vi "PrefDialog.vi"(8 "error in (no error)":errorcluster, 11 "MyPluginsBase in":refnum<class "ChromaPowerSupply.lvclass">) -> (0 "error out":errorcluster, 1 "Save As":bool, 2 "Changed":bool, 3 "MyPluginsBase out":refnum<class "ChromaPowerSupply.lvclass">)   [LabVIEW 2018, in "AcPwrPlugins.lvlib" / "ChromaPowerSupply.lvclass"]
doc: "This VI displays the prior instruments properties and allows a user to change the instrument properties and save these new set properties to the same location on disk or in a new location with a new name called \"Type\"."
uses:
  ChromaPowerSupply.lvclass
  C:/Program Files (x86)/National Instruments/LabVIEW 2018/user.lib/NIST/BaseClasses/BasePlugin_class/BasePlugin.lvclass
  C:/Users/Public/Projects/ICDAS/NistPluggableModules/AcPwr/AcPwrPlugins/AcPwrBaseClass/AcPwrBase.lvclass
  TypeDefs/Measurements.ctl
  AcPwrBaseClass/TypeDefs/BaseMeasurements.ctl
  ChromaAcLoad/TypeDefs/MeasurementType.ctl
  TypeDefs/Device(s)Settings.ctl
  <userlib>/NIST/BaseClasses/BasePlugin_class/BasePlugin.lvclass/BasePlugin.ctl
  AcPwrBaseClass/AcPwrBase.lvclass/AcPwrBase.ctl
  <userlib>/NIST/BaseClasses/BasePlugin_class/Accessors/Read PluginIniFilePath.vi
  AcPwrBaseClass/Accessors/Read BaseConfig.vi
  AcPwrBaseClass/Accessors/Read BaseMeasurements.vi
  <userlib>/NIST/BaseClasses/BasePlugin_class/Accessors/Write PluginIniFilePath.vi
  <vilib>/Utility/config.llb/NI_LVConfig.lvlib
  AcPwrBaseClass/AcPwrBase.lvclass
  ChromaAcLoad/ChromaAcLoad.lvclass
panel:
  in  "btnSaveAs":bool
  in  "btnSave":bool
  in  "Measurement RefreshTime (ms)":u32
  in  "Device(s)Settings":T1
  in  "BaseMeasurements":T2 {"NHRGridSim Phase" items=["All", "A Phase", "B Phase", "C Phase"]; "NHRDC Measurement Type" items=["Voltage"=1, "Positive Peak Voltage"=2, "Positive Peak Voltage Last Fetch"=4, "Negative Peak Voltage"=8, "Negative Peak Voltage Last Fetch"=16, "Current"=32, "Positive Peak Current"=64, "Positive Peak Current Last Fetch"=128, "Negative Peak Current"=256, "Negative Peak Current Last Fetch"=512, "Power"=1024, "Positive Peak Power"=2048, "Positive Peak Power Last Fetch"=4096, "Negative Peak Power"=8192, "Negative Peak Power Last Fetch"=16384, "Timestamp"=32768, "Charge Time"=65536, "Discharge Time"=131072, "Amp Hour"=262144, "Amp Hour Time"=524288, "Amp Hour Charge"=1048576, "Amp Hour Discharge"=2097152, "Kilo Watt Hour"=4194304, "Kilo Watt Hour Time"=8388608, "Kilo Watt Hour Charge"=16777216, "Kilo Watt Hour Discharge"=33554432, "UUT Temperature"=67108864]; "NHRDC Fetch Method" items=["Aperture", "Immediate"]}
  in  "Measurements":T4
  in  "btnCancel":bool
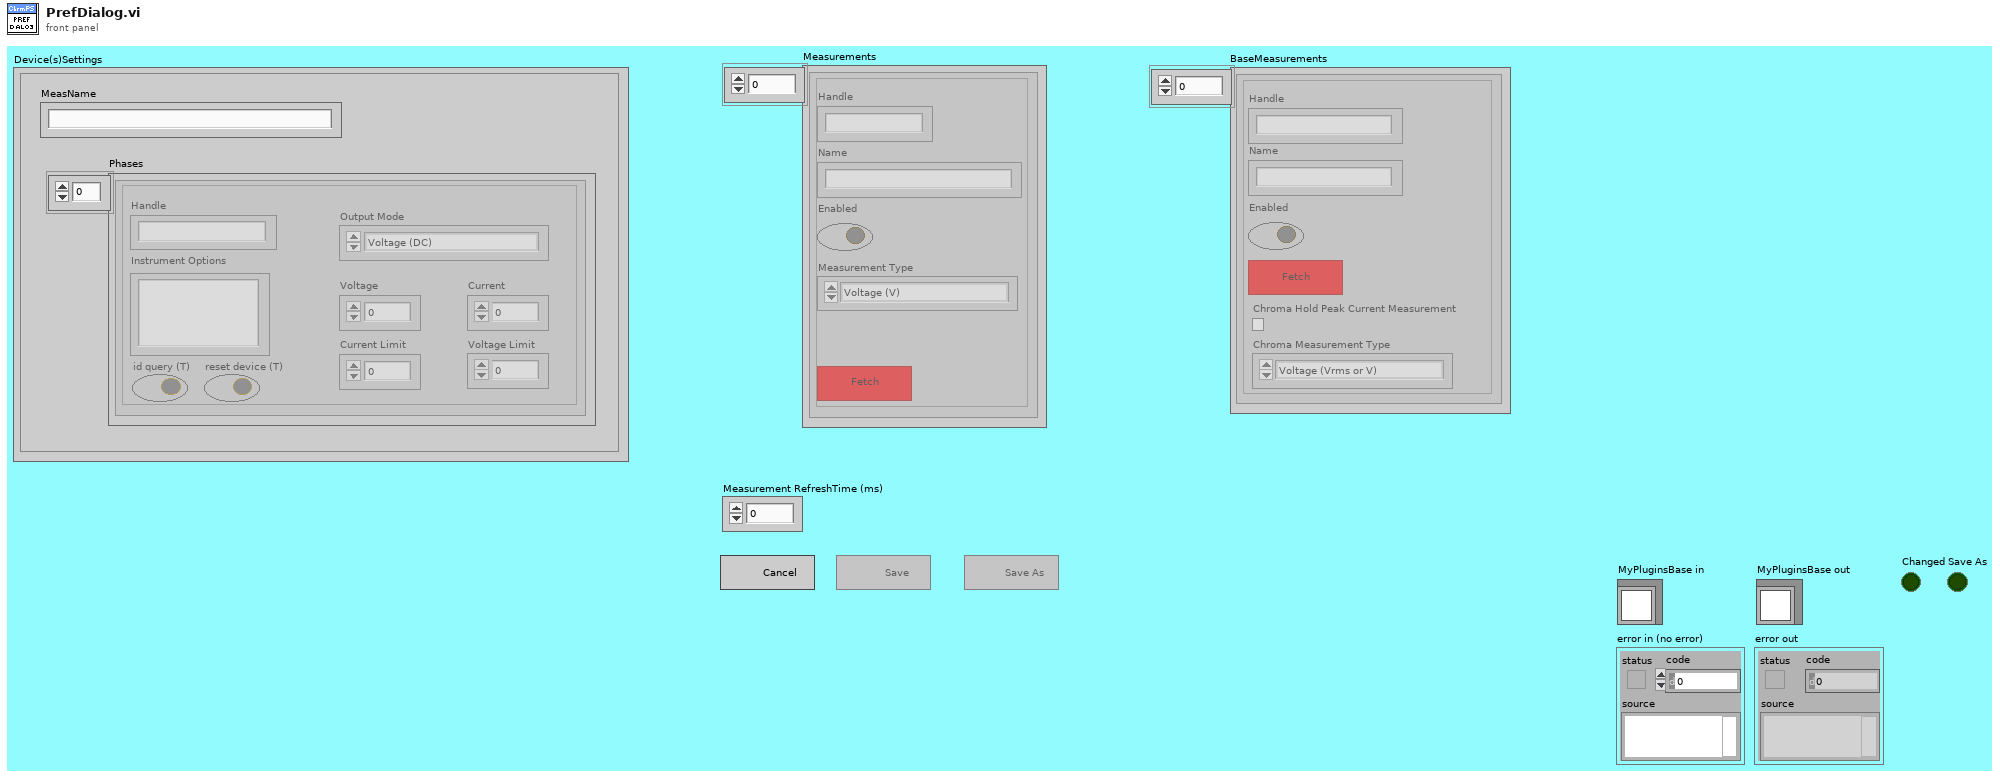
[diagram p1: front panel]
types:
  T1 = typedef "AcPwrPlugins.lvlib/ChromaPowerSupply.lvclass/Device(s)Settings.ctl" = cluster{"Phases":cluster{"Handle":string, "Instrument Options":string, "id query (T)":bool, "reset device (T)":bool, "Timing":cluster{"TimingOn":enum16{""}, "Hours":u32, "Minutes":u32, "Seconds":dbl, "CutoffVoltage":dbl}, "Connected":bool, "Output Mode":enum16{"Voltage (DC)", "Current (DC)"}, "Voltage":dbl, "Current":dbl, "Voltage Limit":dbl, "Current Limit":dbl}[], "MeasName":string}
  T2 = typedef "AcPwrPlugins.lvlib/AcPwrBase.lvclass/BaseMeasurements.ctl" = cluster{"Handle":string, "Name":string, "Enabled":bool, "Measurement Value":dbl, "btnMeasFetch":bool, "Chroma Hold Peak Current Measurement":bool, "Chroma Measurement Type":T3, "Chroma Protection Status String":string, "NHRDC Fetch Method":i32, "NHRDC Fetch Time (s)":sgl, "NHRDC Measurement Type":i32, "NHRGridSim Measurement Type ":enum16{"Average Current", "Max Current", "Min Current", "Average Voltage", "Max Voltage", "Min Voltage", "Average True Power", "Max True Power", "Min True Power", "Average Apparent Power", "Max Apparent Power", "Min Apparent Power", "Power Factor", "Crest Factor"}, "NHRGridSim Phase ":i32, "PPS Measurement Type ":enum16{"Voltage RMS L-N", "Voltage RMS L-L", "Frequency", "Current RMS", "Current Peak", "Crest Factor", "Power Factor", "Power VA", "Real Power"}, "PPS Channel Name":enum16{"A", "B", "C"}}[]
  T3 = typedef "AcPwrPlugins.lvlib/ChromaAcLoad.lvclass/MeasurementType.ctl" = enum16{"Voltage (Vrms or V)", "Current (Arms or A)", "Power (W)", "Peak Voltage (V)", "Peak Current (A)", "Peak Power (W)", "Frequency (Hz)", "Resistance (Ohms)", "Voltage Overshoot (V)", "Positive Peak Current (A)", "Voltage Undershoot (V)", "Negative Peak Current (A)", "Apparent Power (VA)", "Reacitive Power (VAR)", "Voltage THD", "Power Factor", "Current's Crest Factor"}
  T4 = typedef "AcPwrPlugins.lvlib/ChromaPowerSupply.lvclass/Measurements.ctl" = cluster{"Handle":string, "Name":string, "Enabled":bool, "Measurement Value":dbl, "btnMeasFetch":bool, "ProtectionStatusString":string, "Measurement Type":enum16{"Voltage (V)", "Current (A)", "Power (W)"}}[]
  T5 = enum32{"Invalid", "Default", "Floating", "Floating/Auto-Hide", "Modal"}
  T6 = enum32{"Invalid", "Standard", "Closed", "Hidden", "Minimized", "Maximized"}
  T7 = enum8{"Enabled", "Disabled", "Disabled and Grayed Out"}
  T8 = cluster{"Handle":string, "Instrument Options":string, "id query (T)":bool, "reset device (T)":bool, "Timing":cluster{"TimingOn":enum16{""}, "Hours":u32, "Minutes":u32, "Seconds":dbl, "CutoffVoltage":dbl}, "Connected":bool, "Output Mode":enum16{"Voltage (DC)", "Current (DC)"}, "Voltage":dbl, "Current":dbl, "Voltage Limit":dbl, "Current Limit":dbl}[]
  T9 = cluster{"Handle":string, "Instrument Options":string, "id query (T)":bool, "reset device (T)":bool, "Timing":cluster{"TimingOn":enum16{""}, "Hours":u32, "Minutes":u32, "Seconds":dbl, "CutoffVoltage":dbl}, "Connected":bool, "Output Mode":enum16{"Voltage (DC)", "Current (DC)"}, "Voltage":dbl, "Current":dbl, "Voltage Limit":dbl, "Current Limit":dbl}
  T10 = typedef "AcPwrPlugins.lvlib/AcPwrBase.lvclass/BaseConfig.ctl" = cluster{"Frequency":dbl, "FrequencyRange":dbl[], "Phases":T11[], "Name":string, "PluginConfigVariant":variant, "PluginMeasVariant":variant}
  T11 = typedef "AcPwrPlugins.lvlib/AcPwrBase.lvclass/Phase.ctl" = cluster{"Name":string, "Enabled":bool, "VoltageLevel":dbl, "Handle":string, "VoltageRange":dbl[], "Connected":bool, "CurrentLimit":dbl, "Waveform":string}
  T12 = typedef "NI_LVConfig.lvlib/Config Data RefNum.ctl" = refnum<k1>
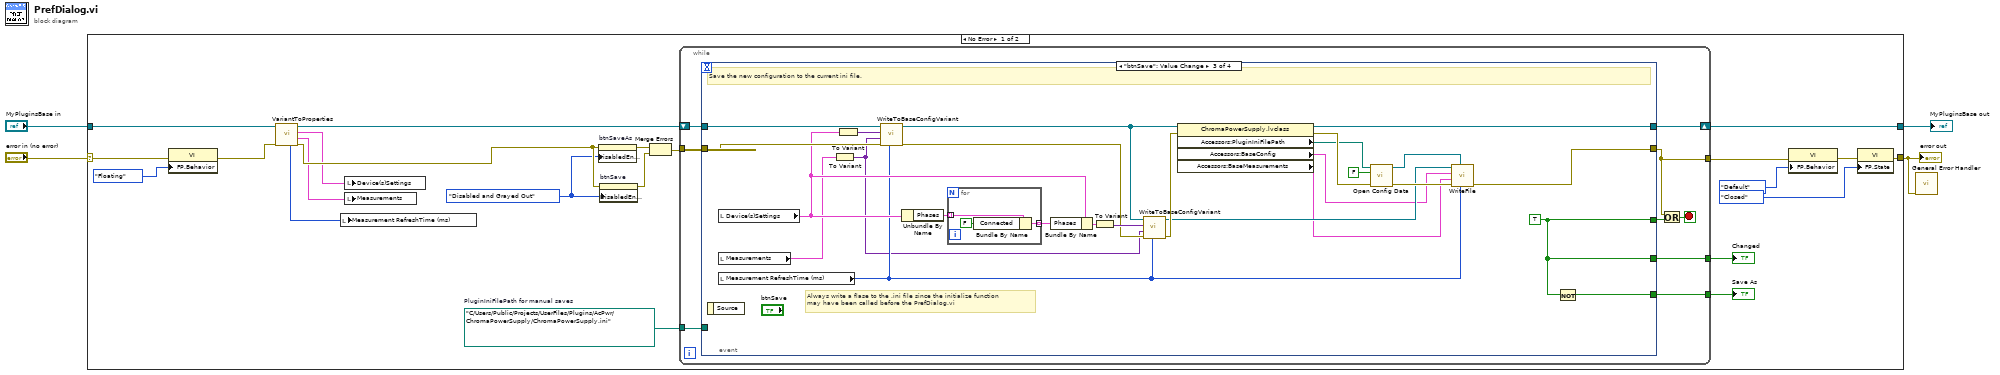
[diagram p0: block diagram]
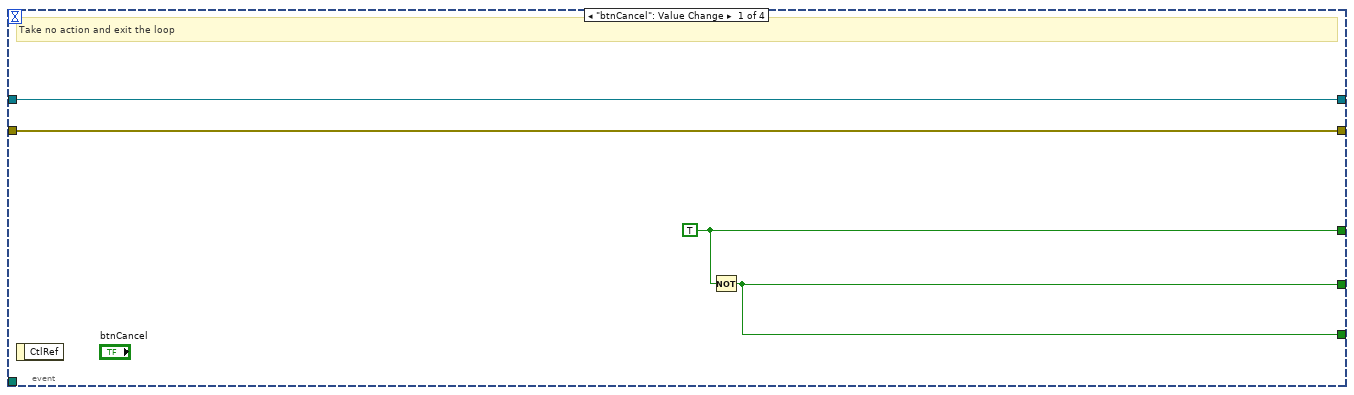
[diagram p2: hidden frame]
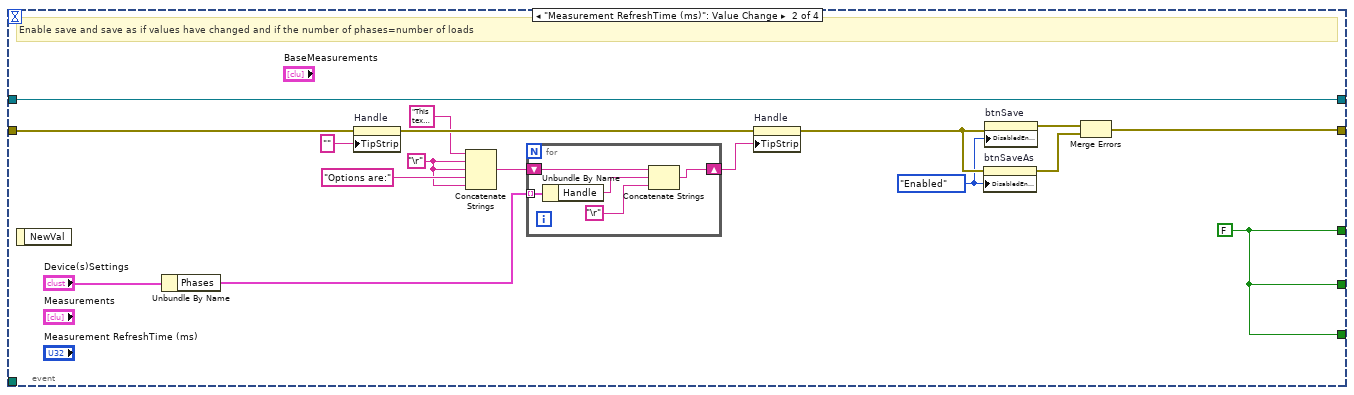
[diagram p3: hidden frame]
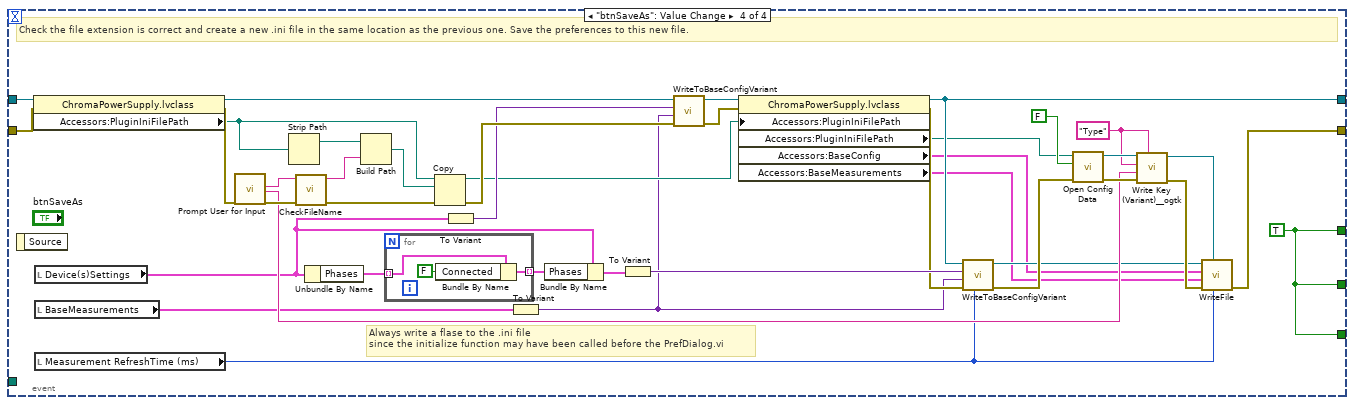
[diagram p4: hidden frame]
diagram:
  n1 = case shown="No Error" "error in (no error)" {
    selector: "error in (no error)" -> [w19 w134]
    tunnel: [w26 w135] -> w2
    tunnel: [w22 w134] -> w1
    tunnel: "MyPluginsBase in" -> [w21 w135]
    frame No Error {
      w11 = T7."Disabled and Grayed Out" ("Disabled")
      w5 = path "C:/Users/Public/Projects/UserFiles/Plugins/AcPwr/ChromaPowerSupply/ChromaPowerSupply.ini"  # PluginIniFilePath for manual saves
      n2 = property class="VI"(error in=w19, "FP.Behavior"=T5."Floating" ("Front Panel Window:Behavior")) -> (error out=w17:errorcluster)  [unwired: 1 in, 1 out]
      n3 = call-dynamic "VariantToProperties.vi"("error in (no error)"=w17, "ChromaPowerSupply in"=w21) -> ("error out"=w15:errorcluster, "Measurements"=w8:T4, "Device Settings"=w10:T1, "ChromaPowerSupply out"=w14:refnum<class "ChromaPowerSupply.lvclass">, "Measurement Refresh Time (ms)"=w9:u32)  [unwired: 5 in]
      n4 = local write "Measurement RefreshTime (ms)"(w9) -> ()
      n5 = local write "Device(s)Settings"(w10) -> ()
      n6 = local write "Measurements"(w8) -> ()
      n7 = property on="btnSaveAs" class="Bool"(error in=w15, "DisabledEnum"=w11) -> (error out=w12:errorcluster)  [unwired: 1 in, 1 out]
      n8 = property on="btnSave" class="Bool"(error in=w15, "DisabledEnum"=w11) -> (error out=w13:errorcluster)  [unwired: 1 in, 1 out]
      n9 = Merge Errors(w12, w13) -> (w16:errorcluster)
      n10 = while {
        shift-right: [w34] -> w26
        shift-left: w14 -> [w35]
        tunnel: w16 -> [w33]
        tunnel: [w29] -> w20
        tunnel: [w32] -> w7
        tunnel: [w31] -> w6
        tunnel: w5 -> [w27]
        stop <- w30 stop-if-true
        n11 = event shown="[2] \"btnSave\": Value Change" {
          selector: _ -> [_ _ _ _]
          dyn-events: _ -> [_ _ _ _]
          timeout: _ -> [_ _ _ _]
          tunnel: w35 -> [w39 w54 w78 w118]
          tunnel: [w37 w55 w85 w124] -> w28
          tunnel: [w39 w54 w70 w98] -> w34
          tunnel: w33 -> [w38 w50 w77 w117]
          tunnel: [w38 w56 w79 w111] -> w29
          tunnel: [w36 w55 w85 w124] -> w32
          tunnel: [w36 w55 w84 w124] -> w31
          tunnel: w27 -> [_ _ _ _]
          event "btnCancel": Value Change {
            w37 = TRUE
            # "Take no action and exit the loop"
            n12 = event-data() -> ()  [unwired: 1 in, 1 out]
            n13 = Not(x=w37) -> (.not. x?=w36:bool)
          }
          event "Measurement RefreshTime (ms)": Value Change {
            w40 = T7."Enabled" ("Disabled")
            w46 = "\r"
            w55 = FALSE
            # "Enable save and save as if values have changed and if the number of phases=number of loads"
            n14 = event-data() -> ()  [unwired: 1 in, 1 out]
            n15 = Unbundle By Name("Device(s)Settings") -> ("Phases"=w43:T8)
            n16 = property on="Handle" class="Str"(error in=w50, "TipStrip"="" ("Tip Strip")) -> (error out=w52:errorcluster)  [unwired: 1 in, 1 out]
            n17 = Concatenate Strings("This text in this handle of the instrument and entered in the  \nhandle control in the Phases array EXACTLY, lest the attempt \nto interact with the instrument will fail.", w46, w46, "Options are:" ("Handle"), w46) -> (w51:string)
            n18 = for {
              shift-right: [w61] -> w53
              shift-left: w51 -> [w60]
              tunnel: w43 -> [w59] mode=indexing
              n19 = Unbundle By Name(w59) -> ("Handle"=w58:string)
              n20 = Concatenate Strings(w60, w58, "\r") -> (w61:string)
            }
            n21 = property on="Handle" class="Str"(error in=w52, "TipStrip"=w53) -> (error out=w44:errorcluster)  [unwired: 1 in, 1 out]
            n22 = property on="btnSaveAs" class="Bool"(error in=w44, "DisabledEnum"=w40) -> (error out=w42:errorcluster)  [unwired: 1 in, 1 out]
            n23 = property on="btnSave" class="Bool"(error in=w44, "DisabledEnum"=w40) -> (error out=w41:errorcluster)  [unwired: 1 in, 1 out]
            n24 = Merge Errors(w41, w42) -> (w56:errorcluster)
          }
          event "btnSave": Value Change {
            w85 = TRUE
            # "Always write a flase to the .ini file since the initialize function\nmay have been called before the PrefDialog.vi"
            # "Save the new configuration to the current ini file."
            n25 = event-data() -> ()  [unwired: 1 in, 1 out]
            n26 = local read "Device(s)Settings"() -> (w68:T1)
            n27 = local read "Measurements"() -> (w64:T4)
            n28 = local read "Measurement RefreshTime (ms)"() -> (w66:u32)
            n29 = To Variant(anything=w64) -> (Variant=w65:variant)
            n30 = To Variant(anything=w68) -> (Variant=w76:variant)
            n31 = call-dynamic "WriteToBaseConfigVariant.vi"("Measurement Refresh Time (ms)"=w66, "error in (no error)"=w77, "Meas"=w65, "Config"=w76, "ChromaPowerSupply in"=w78) -> ("error out"=w72:errorcluster, "ChromaPowerSupply out"=w73:refnum<class "ChromaPowerSupply.lvclass">)  [unwired: 5 in]
            n32 = Unbundle By Name(w68) -> ("Phases"=w83:T8)
            n33 = for {
              tunnel: w83 -> [w89] mode=indexing
              tunnel: [w90] -> w82 mode=indexing
              n34 = Bundle By Name(cluster=w89, "Connected"=FALSE) -> (w90:T9)
            }
            n35 = Bundle By Name(cluster=w68, "Phases"=w82) -> (w74:T1)
            n36 = To Variant(anything=w74) -> (Variant=w75:variant)
            n37 = call-dynamic "WriteToBaseConfigVariant.vi"("Measurement Refresh Time (ms)"=w66, "error in (no error)"=w72, "Meas"=w65, "Config"=w75, "ChromaPowerSupply in"=w73) -> ("error out"=w71:errorcluster, "ChromaPowerSupply out"=w69:refnum<class "ChromaPowerSupply.lvclass">)  [unwired: 5 in]
            n38 = property class="ChromaPowerSupply.lvclass"(reference=w73, error in=w71) -> (reference out=w70:refnum<class "ChromaPowerSupply.lvclass">, error out=w87:errorcluster, "Accessors:PluginIniFilePath"=w62:path, "Accessors:BaseConfig"=w67:T10, "Accessors:BaseMeasurements"=w63:T2)
            n39 = call <vilib>:"Open Config Data.vi"("error in (no error)"=w87, "create file if necessary (T)"=FALSE, "configuration file path"=w62) -> ("error out"=w81:errorcluster, "refnum"=w80:T12)  [unwired: 6 in, 1 out]
            n40 = call-dynamic "WriteFile.vi"("RefreshTime"=w66, "Refnum in"=w80, "error in (no error)"=w81, "BaseMeasurements"=w63, "BaseConfiguration"=w67, "ChromaPowerSupply in"=w69) -> ("error out"=w79:errorcluster)  [unwired: 4 in, 1 out]
            n41 = Not(x=w85) -> (.not. x?=w84:bool)
          }
          event "btnSaveAs": Value Change {
            w125 = "Type" ("section (optional)")
            w124 = TRUE
            # "Always write a flase to the .ini file\nsince the initialize function may have been called before the PrefDialog.vi"
            # "Check the file extension is correct and create a new .ini file in the same location as the previous one. Save the preferences to this new file."
            n42 = event-data() -> ()  [unwired: 1 in, 1 out]
            n43 = property class="ChromaPowerSupply.lvclass"(reference=w118, error in=w117) -> (reference out=w109:refnum<class "ChromaPowerSupply.lvclass">, error out=w116:errorcluster, "Accessors:PluginIniFilePath"=w115:path)
            n44 = local read "Device(s)Settings"() -> (w105:T1)
            n45 = local read "BaseMeasurements"() -> (w93:T2)
            n46 = local read "Measurement RefreshTime (ms)"() -> (w91:u32)
            n47 = call "Prompt User for Input"("error in (no error)"=w116) -> ("File Name"=w119:string, "PluginType"=w122:string, "error out"=w123:errorcluster)  [unwired: 15 in, 1 out]
            n48 = Strip Path(path=w115) -> (stripped path=w129:path)  [unwired: 1 out]
            n49 = call "CheckFileName.vi"("Error In"=w123, "File Name in"=w119) -> ("Error Out"=w121:errorcluster, "File Name out"=w120:string)  [unwired: 8 in]
            n50 = Unbundle By Name(w105) -> ("Phases"=w114:T8)
            n51 = Build Path(base path=w129, name or relative path=w120) -> (appended path=w128:path)
            n52 = for {
              tunnel: w114 -> [w131] mode=indexing
              tunnel: [w133] -> w113 mode=indexing
              n53 = Bundle By Name(cluster=w131, "Connected"=FALSE) -> (w133:T9)
            }
            n54 = Copy(8:w121, 10:w128, 11:w115) -> (0:w107:errorcluster, 3:w97:path)  [unwired: 2 in, 1 out]
            n55 = To Variant(anything=w105) -> (Variant=w106:variant)
            n56 = To Variant(anything=w93) -> (Variant=w92:variant)
            n57 = Bundle By Name(cluster=w105, "Phases"=w113) -> (w104:T1)
            n58 = To Variant(anything=w104) -> (Variant=w103:variant)
            n59 = call-dynamic "WriteToBaseConfigVariant.vi"("error in (no error)"=w107, "Meas"=w92, "Config"=w106, "ChromaPowerSupply in"=w109) -> ("error out"=w108:errorcluster, "ChromaPowerSupply out"=w102:refnum<class "ChromaPowerSupply.lvclass">)  [unwired: 6 in]
            n60 = property class="ChromaPowerSupply.lvclass"(reference=w102, error in=w108, "Accessors:PluginIniFilePath"=w97) -> (reference out=w98:refnum<class "ChromaPowerSupply.lvclass">, error out=w101:errorcluster, "Accessors:PluginIniFilePath"=w96:path, "Accessors:BaseConfig"=w95:T10, "Accessors:BaseMeasurements"=w94:T2)
            n61 = call-dynamic "WriteToBaseConfigVariant.vi"("Measurement Refresh Time (ms)"=w91, "error in (no error)"=w101, "Meas"=w92, "Config"=w103, "ChromaPowerSupply in"=w98) -> ("error out"=w100:errorcluster, "ChromaPowerSupply out"=w99:refnum<class "ChromaPowerSupply.lvclass">)  [unwired: 5 in]
            n62 = call <vilib>:"Open Config Data.vi"("error in (no error)"=w100, "create file if necessary (T)"=FALSE, "configuration file path"=w96) -> ("error out"=w127:errorcluster, "refnum"=w126:T12)  [unwired: 6 in, 1 out]
            n63 = call <userlib>:"Write Key (Variant)__ogtk.vi"("section"=w125, "error in (no error)"=w127, "key-value"=w122, "key (optional)"=w125, "refnum"=w126) -> ("error out"=w112:errorcluster, "refnum out"=w110:T12)  [unwired: 5 in]
            n64 = call-dynamic "WriteFile.vi"("RefreshTime"=w91, "Refnum in"=w110, "error in (no error)"=w112, "BaseMeasurements"=w94, "BaseConfiguration"=w95, "ChromaPowerSupply in"=w99) -> ("error out"=w111:errorcluster)  [unwired: 4 in, 1 out]
          }
        }
        n65 = Or(x=w29, y=w28) -> (x .or. y?=w30:bool)
      }
      "Save As" <- w6
      "Changed" <- w7
      n66 = property class="VI"(error in=w20, "FP.Behavior"=T5."Default" ("Front Panel Window:Behavior")) -> (error out=w25:errorcluster)  [unwired: 1 in, 1 out]
      n67 = property class="VI"(error in=w25, "FP.State"=T6."Closed" ("Front Panel Window:State")) -> (error out=w22:errorcluster)  [unwired: 1 in, 1 out]
    }
    frame Error {
    }
  }
  "error out" <- w1
  "MyPluginsBase out" <- w2
  n68 = call <vilib>:"General Error Handler.vi"("error in (no error)"=w1) -> ()  [unwired: 10 in, 5 out]
